vi "ScriptingTest.vi"() -> ()   [LabVIEW 2018]
doc: "VI for scripting the exposed classes in this example to Python or Matlab"
uses:
  Published Classes/Console_class/Console.lvclass
  Published Classes/PerformanceTest_class/PerformanceTest.lvclass
  Scripting/Matlab_class/Matlab.lvclass
  C:/VIT/VIT-Reuse/Examples/RemoteLabviewInterface/Scripting/Scripting_class/Scripting.lvclass
  Scripting/Python_class/Python.lvclass
  Executer_class/Executer.lvclass
panel:
  in  "Python (t)/ Matlab(f)":bool=TRUE
  out "Error Out":errorcluster
  in  "Output Folder":path=path "C:/VIT/VIT-Reuse/Examples/RemoteLabviewInterface/Scripts/Python"
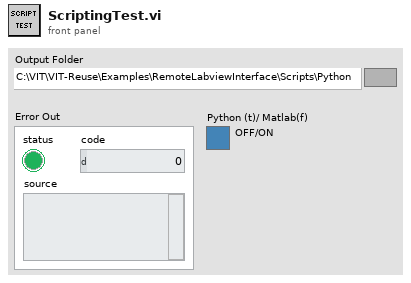
[diagram p1: front panel]
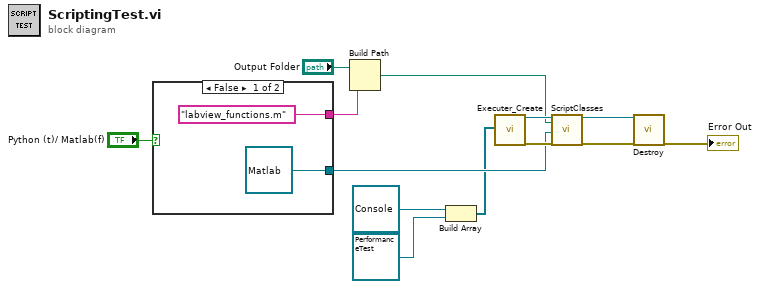
[diagram p0: block diagram]
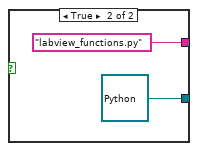
[diagram p2: hidden frame]
diagram:
  n1 = case shown="False" "Python (t)/ Matlab(f)" {
    tunnel: [refnum<class "Matlab.lvclass"> refnum ("Matlab") refnum<class "Python.lvclass"> refnum ("Python")] -> w6
    tunnel: ["labview_functions.m" ("name or relative path") "labview_functions.py" ("name or relative path")] -> w4
    frame False {
    }
    frame True {
    }
  }
  n2 = Build Path(base path="Output Folder", name or relative path=w4) -> (appended path=w3:path)
  n3 = Build Array(refnum<class "Console.lvclass"> refnum ("Console"), refnum<class "PerformanceTest.lvclass"> refnum ("TimingMethods")) -> (w5:refnum<class>[])
  n4 = call "Executer_Create.vi"("Classes"=w5) -> ("reference out"=w13:refnum<class "Executer.lvclass">, "error out"=w11:errorcluster)  [unwired: 17 in]
  n5 = call-dynamic "ScriptClasses.vi"("reference in"=w13, "Filepath"=w3, "Scripting"=w6, "error in (no error)"=w11) -> ("reference out"=w12:refnum<class "Executer.lvclass">, "error out"=w10:errorcluster)  [unwired: 14 in]
  n6 = call-dynamic "Destroy.vi"("reference in"=w12, "error in (no error)"=w10) -> ("error out"=→"Error Out":errorcluster)  [unwired: 16 in, 1 out]
